vi "getIntensity.vi"(6 "Fiber Num":i32, 8 "Error":bool, 9 "VISA resource name":refnum<visa-resource-name>="ASRL13::INSTR") -> (1 "Intensity":dbl, 2 "Error":bool, 3 "dup VISA resource name":refnum<visa-resource-name>="ASRL13::INSTR")   [LabVIEW 2018]
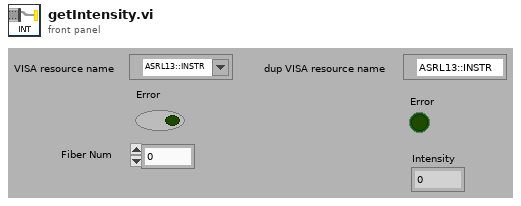
[diagram p1: front panel]
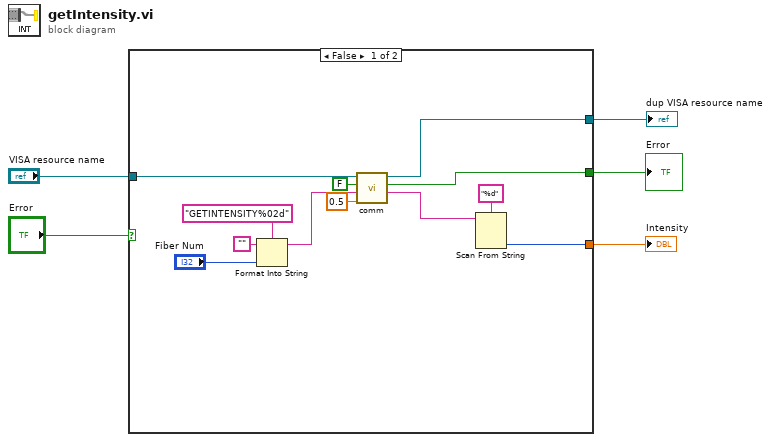
[diagram p0: block diagram]
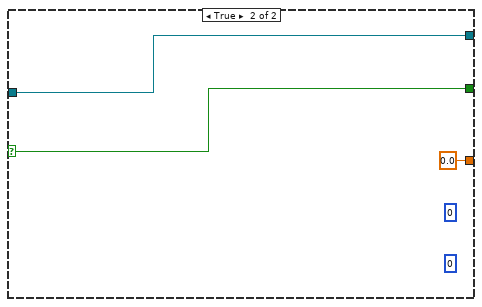
[diagram p2: hidden frame]
diagram:
  n1 = case shown="False" "Error" {
    selector: "Error" -> [_ w20]
    tunnel: "VISA resource name" -> [w17 w19]
    tunnel: [w15 0.0] -> w4
    tunnel: [w10 w19] -> w3
    tunnel: [w9 w20] -> w2
    frame False {
      n2 = Format Into String(format string="GETINTENSITY%02d" ("Substring"), initial string="", "Fiber Num") -> (resulting string=w11:string)  [unwired: 1 in, 1 out]
      n3 = call "comm.vi"("Timeout (s)"=0.5, "Command"=w11, "Error"=FALSE, "VISA resource name"=w17) -> ("Response"=w8:string, "Error"=w9:bool, "dup VISA resource name"=w10:refnum<visa-resource-name>)  [unwired: 2 in, 1 out]
      n4 = Scan From String(format string="%d", input string=w8) -> (output 1=w15:i32)  [unwired: 3 in, 3 out]
    }
    frame True {
      (unwired) 0
      (unwired) 0
    }
  }
  "dup VISA resource name" <- w3
  "Error" <- w2
  "Intensity" <- w4
